vi "Heizungsregler.vi"() -> ()   [LabVIEW 2024]
uses:
  Treiber Heizung/Thermostat Treiber.lvlib
panel:
  out "Temperaturgraph":cluster{timestamp, dbl}[](graph)
  in  "Stop":bool
  in  "Thermostat":i32(knob) scale=0.0..3.0
  # "Heizungsregelung"
  # "Thermostat:\nStufe 0: Regler Aus\nStufe 1: 30°C\nStufe 2: 45°C\nStufe 3: 60°C"
  # "Thermostat"
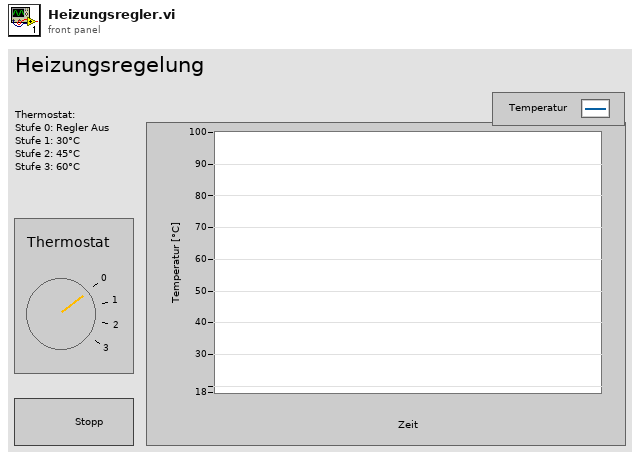
[diagram p1: front panel]
types:
  T1 = cluster{"Zeitstempel-Bedienelement":timestamp, "Temperatur":dbl}
  T2 = cluster{"Zeitstempel-Bedienelement":timestamp, "Temperatur":dbl}[]
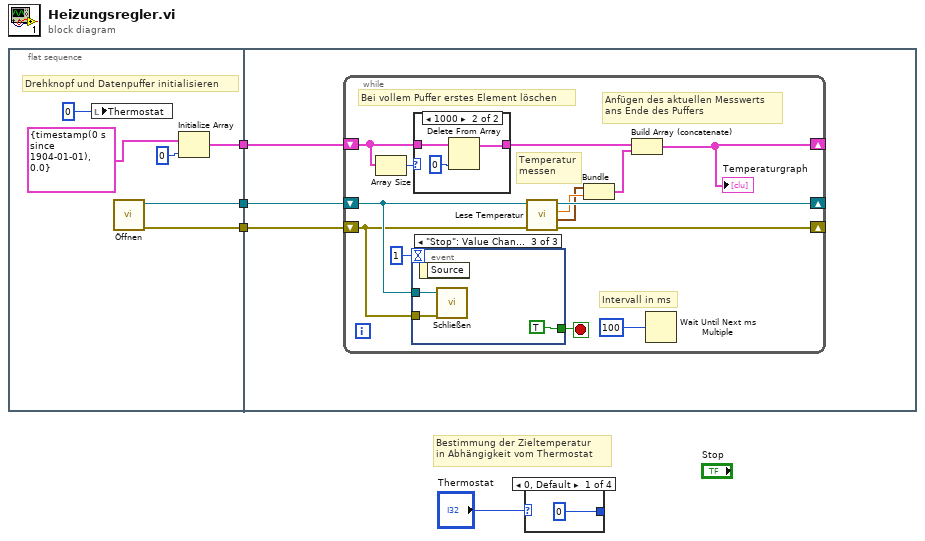
[diagram p0: block diagram]
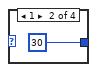
[diagram p2: hidden frame]
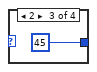
[diagram p3: hidden frame]
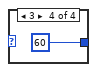
[diagram p4: hidden frame]
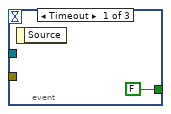
[diagram p6: hidden frame]
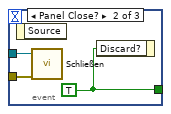
[diagram p7: hidden frame]
diagram:
  # "Bestimmung der Zieltemperatur\nin Abhängigkeit vom Thermostat"
  n1 = flat-sequence {
    tunnel: [w9] -> w4
    tunnel: [w8] -> w3
    tunnel: [w5] -> w1
    tunnel: w4 -> [w13]
    tunnel: w3 -> [w12]
    tunnel: w1 -> [w11]
    frame #0 {
      # "Drehknopf und Datenpuffer initialisieren"
      n2 = local write "Thermostat"(0 ("Knob")) -> ()
      n3 = call "Öffnen.vi"() -> ("Error Out"=w8:errorcluster, "Verbindungs-ID"=w9:refnum<k16>)  [unwired: 10 in]
      n4 = Initialize Array(cluster{timestamp, dbl} {timestamp(0 s since 1904-01-01), 0.0}, 0 ("dimension size")) -> (w5:cluster{timestamp, dbl}[])
    }
    frame #1 {
      n5 = while {
        shift-right: [w24] -> _
        shift-left: w13 -> [w25]
        shift-right: [w23] -> _
        shift-left: w12 -> [w22]
        shift-right: [w14] -> _
        shift-left: w11 -> [w16]
        stop <- w27 stop-if-true
        # "Anfügen des aktuellen Messwerts\nans Ende des Puffers"
        # "Temperatur\nmessen"
        # "Bei vollem Puffer erstes Element löschen"
        # "Intervall in ms"
        n6 = Array Size(array=w16) -> (size(s)=w18:i32)
        n7 = event shown="[2] \"Stop\": Value Change" {
          selector: _ -> [_ _ _]
          dyn-events: _ -> [_ _ _]
          timeout: 1 -> [_ _ _]
          tunnel: [FALSE ("Discard?") w35 TRUE ("Discard?")] -> w27
          tunnel: w25 -> [_ w34 w37]
          tunnel: w22 -> [_ w33 w36]
          event Timeout {
            n8 = event-data() -> ()  [unwired: 1 in, 1 out]
          }
          event Panel Close? {
            w35 = TRUE ("Discard?")
            n9 = event-data() -> ()  [unwired: 1 in, 1 out]
            n10 = call "Schließen.vi"("Error In"=w33, "Verbindungs-ID"=w34) -> ()  [unwired: 9 in, 1 out]
            n11 = event-data("Discard?"=w35) -> ()  [unwired: 1 in, 1 out]
          }
          event "Stop": Value Change {
            n12 = event-data() -> ()  [unwired: 1 in, 1 out]
            n13 = call "Schließen.vi"("Error In"=w36, "Verbindungs-ID"=w37) -> ()  [unwired: 9 in, 1 out]
          }
        }
        n14 = case shown="1000" w18 {
          tunnel: w16 -> [w28 w31]
          tunnel: [w28 w30] -> w15
          frame 0, Default {
          }
          frame 1000 {
            n15 = Delete From Array(array=w31, index=0) -> (array with subset deleted=w30:cluster{timestamp, dbl}[])  [unwired: 1 in, 1 out]
          }
        }
        n16 = call "Lese Temperatur.vi"("Error In"=w22, "Verbindungs-ID in"=w25) -> ("Error Out"=w23:errorcluster, "Zeitstempel-Bedienelement"=w20:timestamp, "Temperatur"=w21:dbl, "Verbindungs-ID out"=w24:refnum<k16>)  [unwired: 5 in, 1 out]
        n17 = Bundle("Zeitstempel-Bedienelement"=w20, "Temperatur"=w21) -> (w19:T1)  [unwired: 1 in]
        n18 = Build Array (concatenate)(w15, w19) -> (w14:T2)
        "Temperaturgraph" <- w14
        n19 = Wait Until Next ms Multiple(millisecond multiple=u32 100) -> ()  [unwired: 1 out]
      }
    }
  }
  n20 = case shown="0, Default" "Thermostat" {
    tunnel: [0 30 45 60] -> _
    frame 0, Default {
    }
    frame 1 {
    }
    frame 2 {
    }
    frame 3 {
    }
  }
